vi "testSendTelFromClient.vi"(8 "error in (no error)":errorcluster) -> (0 "error out":errorcluster)   [LabVIEW 2018]
doc: "This VI sends telemetry from TCP client to TCP server."
uses:
  <vilib>/addons/_JKI Toolkits/Caraya/classes/Assert/Assert Equal Value_Variant.vi
  src/TcpServer/TcpServer.lvclass
  <vilib>/addons/_JKI Toolkits/Caraya/classes/Test/Test.lvclass
  <vilib>/addons/_JKI Toolkits/Caraya/classes/Assert/Assert.lvclass
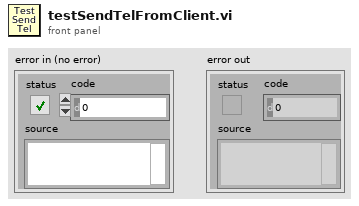
[diagram p1: front panel]
types:
  T1 = cluster{"CmdRead":refnum<user-event>, "EvtRead":refnum<user-event>, "GenRead":refnum<user-event>}
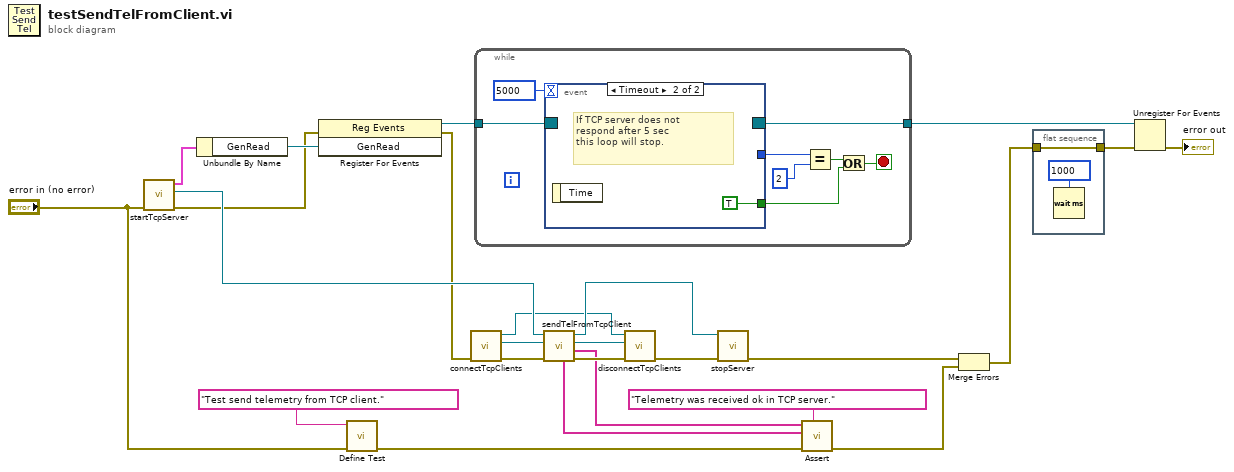
[diagram p0: block diagram]
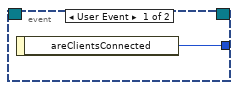
[diagram p2: hidden frame]
diagram:
  n1 = call "startTcpServer.vi"("error in (no error)"="error in (no error)") -> ("error out"=w9:errorcluster, "TcpServer out"=w12:refnum<class "TcpServer.lvclass">, "UserEvents"=w19:T1)  [unwired: 8 in]
  n2 = Unbundle By Name(w19) -> ("GenRead"=w18:refnum<user-event>)
  n3 = register-events(error in=w9, w18) -> (reference out=w25:refnum<event-registration>, error out=w1:errorcluster)  [unwired: 1 in]
  n4 = call <vilib>:"Define Test.vi"("error in (no error)"="error in (no error)", "Label (VI Title)"="Test send telemetry from TCP client.") -> ("error out"=w16:errorcluster)  [unwired: 9 in]
  n5 = call "connectTcpClients.vi"("error in (no error)"=w1) -> ("error out"=w10:errorcluster, "tel connection ID out"=w7:refnum<k5>, "cmd connection ID out"=w8:refnum<k5>)  [unwired: 8 in]
  n6 = while {
    tunnel: w25 -> [w33]
    tunnel: [w32] -> w24
    stop <- w29 stop-if-true
    n7 = event shown="[1] Timeout" {
      selector: w33 -> [_ _]
      dyn-events: [_ _] -> w32
      timeout: 5000 -> [_ _]
      tunnel: [w34 _] -> w31
      tunnel: [_ TRUE] -> w26
      event User Event {
        n8 = event-data() -> ("areClientsConnected"=w34:enum16{"unchanged", "connected", "unconnected"})  [unwired: 1 in]
      }
      event Timeout {
        # "If TCP server does not\nrespond after 5 sec\nthis loop will stop."
        n9 = event-data() -> ()  [unwired: 1 in, 1 out]
      }
    }
    n10 = Equal?(x=w31, y=2) -> (x = y?=w27:bool)
    n11 = Or(x=w27, y=w26) -> (x .or. y?=w29:bool)
  }
  n12 = call "sendTelFromTcpClient.vi"("error in (no error)"=w10, "tel connection ID in"=w7, "TcpServer in"=w12) -> ("error out"=w5:errorcluster, "telemetry sent"=w3:string[], "tel connection ID out"=w6:refnum<k5>, "TcpServer out"=w11:refnum<class "TcpServer.lvclass">, "telemetry received"=w2:string[])  [unwired: 4 in]
  n13 = call "disconnectTcpClients.vi"("error in (no error)"=w5, "tel connection ID in"=w6, "cmd connection ID in"=w8) -> ("error out"=w4:errorcluster)  [unwired: 8 in]
  n14 = call "stopServer.vi"("error in (no error)"=w4, "tcpServer in"=w11) -> ("error out"=w22:errorcluster)  [unwired: 8 in, 1 out]
  n15 = call-poly <vilib>:"Assert.vi"("Label"="Telemetry was received ok in TCP server.", "error in (no error)"=w16, "Y"=w2, "X"=w3) -> ("error out"=w13:errorcluster)  [unwired: 7 in]
  n16 = Merge Errors(w22, w13) -> (w14:errorcluster)
  n17 = flat-sequence {
    tunnel: w14 -> [w36]
    tunnel: [w36] -> w21
    frame #0 {
      n18 = Wait (ms)(milliseconds to wait=u32 1000) -> ()  [unwired: 1 out]
    }
  }
  n19 = Unregister For Events(event registration refnum=w24, error in=w21) -> (error out=→"error out":errorcluster)
